vi "PVCamPropertyChangedCallbackForCameraState.vi"(4 "?":refnum<vi>, 5 "Event Data":cluster{"sender":refnum<k24>, "e":refnum<k24>}, 6 "Control Ref":refnum<k24>, 7 "Event Common Data":T1) -> ()   [LabVIEW 2019]
uses:
  Dependencies/PVCamNET.dll
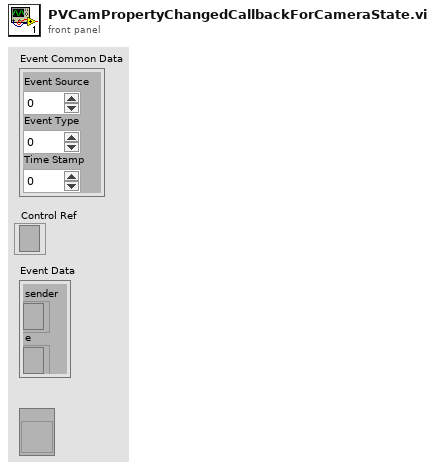
[diagram p1: front panel]
types:
  T1 = cluster{"Event Source":i32, "Event Type":u32, "Time Stamp":u32}
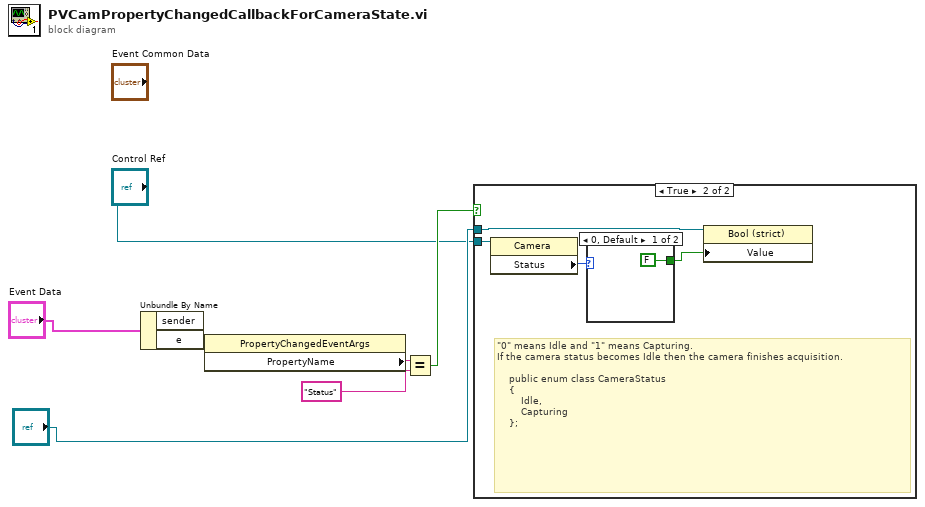
[diagram p0: block diagram]
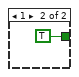
[diagram p3: hidden frame]
diagram:
  n1 = Unbundle By Name("Event Data") -> ("e"=w7:refnum<k24>)  [unwired: 1 out]
  n2 = property class="PropertyChangedEventArgs"(reference=w7) -> ("PropertyName"=w6:string)  [unwired: 1 in, 2 out]
  n3 = Equal?(x=w6, y="Status") -> (x = y?=w4:bool)
  n4 = case shown="True" w4 {
    tunnel: "?" -> [_ w9]
    tunnel: "Control Ref" -> [_ w11]
    frame False {
    }
    frame True {
      # "\"0\" means Idle and \"1\" means Capturing.\nIf the camera status becomes Idle then the camera finishes acquisition.\n\n    public enum class CameraStatus\n    {\n        Idle,\n        Capturing\n    };"
      n5 = property class="Camera"(reference=w11) -> ("Status"=w10:i32)  [unwired: 1 in, 2 out]
      n6 = case shown="0, Default" w10 {
        tunnel: [FALSE TRUE] -> w8
        frame 0, Default {
        }
        frame 1 {
        }
      }
      n7 = property class="Bool (strict)"(reference=w9, "Value"=w8) -> ()  [unwired: 1 in, 2 out]
    }
  }
